vi "Set X Y and Cost.vi"(8 "Cost":dbl, 9 "y":i32, 10 "x":i32, 11 "OccupancyGridMapNode in":refnum<class "NI_Robotics_OccupancyGridMapNode.lvclass">) -> (3 "OccupancyGridMapNode out":refnum<class "NI_Robotics_OccupancyGridMapNode.lvclass">)   [LabVIEW 2017, in "NI_Robotics_OccupancyGridMapNode.lvclass"]
uses:
  <vilib>/robotics/Navigation/shared/MapNode/OccupancyGridNode/NI_Robotics_OccupancyGridMapNode.lvclass
  <vilib>/robotics/Navigation/shared/MapNode/OccupancyGridNode/NI_Robotics_OccupancyGridMapNode.lvclass/NI_Robotics_OccupancyGridMapNode.ctl
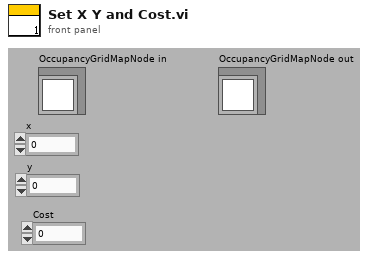
[diagram p1: front panel]
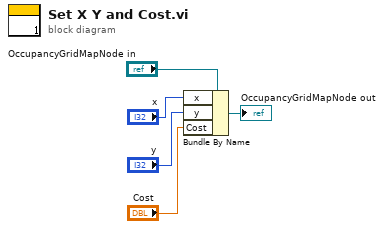
[diagram p0: block diagram]
diagram:
  n1 = Bundle By Name(cluster="OccupancyGridMapNode in", "x"="x", "y"="y", "Cost"="Cost") -> (→"OccupancyGridMapNode out":refnum<class "NI_Robotics_OccupancyGridMapNode.lvclass">)
